vi "Clear_Info.vi"(8 "error in (no error)":errorcluster, 9 "index in":string, 10 "buildObject":T1, 11 "IB_Shortcut in":refnum<class "IB_Shortcut.lvclass">) -> (0 "error out":errorcluster, 1 "index out":string, 2 "buildObject out":T1, 3 "IB_Shortcut out":refnum<class "IB_Shortcut.lvclass">)   [LabVIEW 2020, in "IB_Shortcut.lvclass"]
uses:
  <vilib>/AppBuilder/IB_Classes/Shortcut/IB_Shortcut.lvclass
  <vilib>/AppBuilder/IB_Classes/Shortcut/IB_Shortcut.lvclass/IB_Shortcut.ctl
  <vilib>/AppBuilder/IB_RW_Project/IB_RW_Project_PropBag_Action.ctl
  <resource>/Framework/Providers/API/ItemRef.ctl
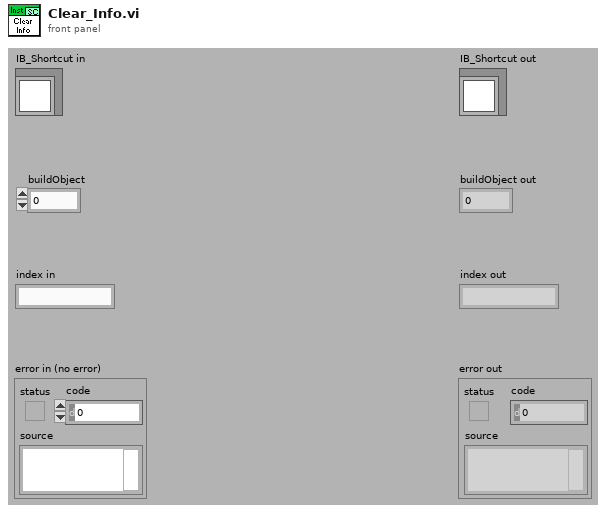
[diagram p1: front panel]
types:
  T1 = typedef "ItemRef.ctl" = u64
  T2 = typedef "IB_RW_Project_PropBag_Action.ctl" = enum16{"read", "write", "clear", "readPrevious", "writePrevious", "clearPrevious"}
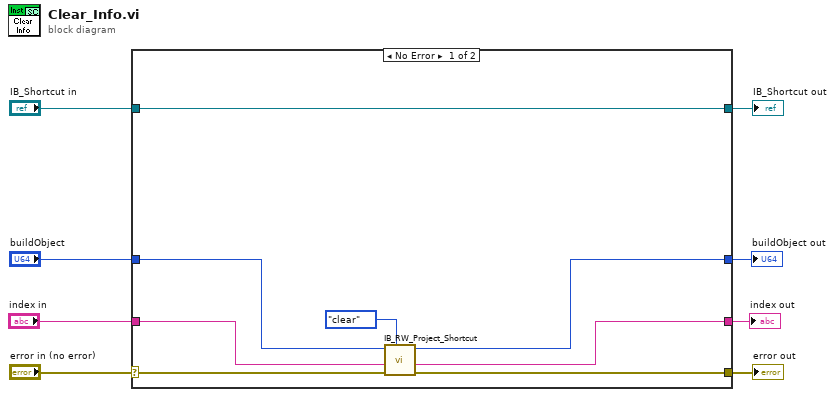
[diagram p0: block diagram]
diagram:
  n1 = case shown="No Error" "error in (no error)" {
    selector: "error in (no error)" -> [w14 w20]
    tunnel: [w13 w20] -> w7
    tunnel: [w16 w19] -> w5
    tunnel: "IB_Shortcut in" -> [w16 w19]
    tunnel: "buildObject" -> [w12 w18]
    tunnel: [w11 w18] -> w3
    tunnel: [w10 w17] -> w2
    tunnel: "index in" -> [w9 w17]
    frame No Error {
      n2 = call <vilib>:"IB_RW_Project_Shortcut.vi"("action"=IB_RW_Project_PropBag_Action."clear", "error in (no error)"=w14, "index in"=w9, "buildObject"=w12) -> ("error out"=w13:errorcluster, "index out"=w10:string, "buildObject out"=w11:T1)  [unwired: 4 in, 1 out]
    }
    frame Error {
    }
  }
  "error out" <- w7
  "IB_Shortcut out" <- w5
  "buildObject out" <- w3
  "index out" <- w2
